vi "AlliGator Send Local Decay Plots.vi"(8 "error in (no error)":errorcluster, 10 "ROI Descriptor":T1 {"Contours"."Type" items=["No Selection", "Point", "Line", "Rectangle", "Oval", "Polygon", "Freehand Region", "Annulus", "Unused2", "Unused3", "Broken Line", "Freehand Line", "Rotated Rectangle"]}, 11 "AlliGator IV DVR in":refnum<data-value>) -> (0 "error out":errorcluster, 3 "AlliGator IV DVR out":refnum<data-value>)   [LabVIEW 2021, in "AlliGator Local Decay Window.lvlib"]
doc: "Gets the data (decay, fit, IRF, residuals and fit parameters) at the selected ROI and sends it to the Local Decay Window for update."
uses:
  AlliGator Local Decay Window.lvlib
  AlliGator Internal Variables v2.ctl
  <vilib>/vision/Image Controls.llb/IMAQ Image.ctl
  AlliGator Gate Image Set.ctl
  AlliGator FLI Dataset Type.ctl
  AlliGator Data Series Type.ctl
  AlliGator Dataset Channel.ctl
  AlliGator Gate Arithmetic.ctl
  AlliGator Displayed Image.ctl
  Image/Named ROI Description.ctl
  AlliGator Decay Metadata v3.ctl
  AlliGator Decay Background Subtraction Info.ctl
  AlliGator Baseline Subtraction Method.ctl
  Graphs/XY Graph/XY Graph Plot Shift Parameters.ctl
  Graphs/XY Graph/XY Graph Plot Shift Method.ctl
  AlliGator Decay Extrapolation Parameters.ctl
  Phasor/Calibration Phasor (m, phi).ctl
  Phasor/Phasor Reference Series.ctl
  Phasor/Phasor Calibration Map v2.ctl
  Phasor/Phasor (g, s).ctl
  AlliGator Raw Phasor Plot Data v4.ctl
  Phasor/Phasor Standard Deviation Options.ctl
  AlliGator Phasor Multi-Harmonic Data.ctl
  Phasor/Phasor Harmonic Data.ctl
  AlliGator Decay Fit Options & Parameters v2.ctl
  Fits/IRF(X)PSED/Decay Fit Options v2.ctl
  Fits/Decay Convolution/Decay Model.ctl
  Fits/Residual Type.ctl
  Fits/IRF(X)PSED/Fit Weights Type.ctl
  Fits/Non-linear Fitting Method v2.ctl
  Fits/Fit Calculation Method.ctl
  Fits/Non-linear Fitting Algorithm.ctl
  AlliGator Decay Fit Parameter Constraints 2.ctl
  Fits/IRF(X)PSED/Decay Fit Parameters In List.ctl
  Fits/IRF(X)PSED/MLE Baseline Offset Type.ctl
  AlliGator Decay Preprocessing Parameters.ctl
  Fits/IRF(X)PSED/Decay Fit Parameters & Derived Quantities List.ctl
  AlliGator Variables List.ctl
  AlliGator Local Decay Graph Window Event Refnum.ctl
  AlliGator Local Decay Fit Results.ctl
  AlliGator Image Profile Plot Data.ctl
  Graphs/XY Graph/XY Plot Data.ctl
  Utilities/Read-Write.ctl
  Variant/Variant to Data/Variant to U16.vi
  Variant/Variant to Data/Variant to Boolean.vi
  AlliGator Globals, Variables & Constants.lvlib
  Graphs/XY Graph/XY Graph Add-Ons.lvlib
  AlliGator Image Profile Window.lvlib
  AlliGator Decay Processing.lvlib
  Time/Time.lvlib
  AlliGator Decay Fit Parameter Map.lvlib
  AlliGator Decay Preprocessing.lvlib
  AlliGator GUI.lvlib
  Utilities/Utilities.lvlib
  Variant/Variant to Data/Variant to Data.lvlib
  Image/Image.lvlib
  Phasor/Phasor.lvlib
  AlliGator Internal Variables.lvlib
  AlliGator Files.lvlib
  AlliGator Phasor Graph.lvlib
  AlliGator Phasor Plot.lvlib
  AlliGator Source Image.lvlib
  Fits/Fits.lvlib
  AlliGator Decay Fit.lvlib
  AlliGator Settings.lvlib
  AlliGator Dual-Channel Datasets.lvlib
panel:
  out "CPU (s)":dbl
  # "see the AlliGator License on the block diagram (Ctrl+E or Window:Show Block Diagram)"
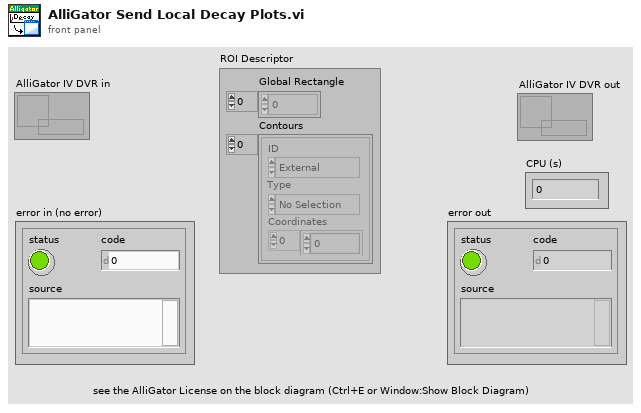
[diagram p1: front panel]
types:
  T1 = typedef "ROI Descriptor" = cluster{"Global Rectangle":i32[], "Contours":cluster{"ID":enum32{"External", "Internal"}, "Type":u32, "Coordinates":i32[]}[]}
  T2 = typedef "AlliGator Local Decay Window.lvlib/AlliGator Local Decay Graph Window Event Refnum.ctl" = refnum<user-event>
  T3 = typedef "AlliGator Globals, Variables & Constants.lvlib/AlliGator Variables List.ctl" = enum16{"---- GUI ----", "Initialization Status", "State Indicators Refnum", "Original AlliGator Menu Items", "Current Action Loop State", "Script in progress", "Playback", "Loop Playback", "Search ROI Used", "Search ROI", "Decay Graph Max Legend Size", "Intensity Graph Max Legend Size", "Decay Statistics Graph Max Legend Size", "Phasor Graph Max Legend Size", "Phasor Ratio Graph Max Legend Size", "Lifetime Graph Max Legend Size", "---- Files ----", "Export Dataset Frames as Individual Files", "Show Batch Export Help Balloons", "Frames in Dataset", "ptu File Frame Start Indices", "Current Frame in Dataset", "Current Frame Timestamp", "------ Python Plugins ------", "Python Plugins Information", "Python Session", "Valid Python Session?", "---- Source Image ----", "Dataset Loaded", "Dataset Metadata", "Dataset Channel", "Dataset Data Description", "Background Dataset Metadata", "Background Dataset Channel", "Background Dataset Data Description", "Background File Subtraction", "Background File Path", "Background File Pile-up Correction", "Background File Pixel Well Capacity", "Background File Scaling Factor", "Source Image ROIs", "Current Source Image ROI", "Source Image ROI Event Refnum", "X_Source Image Display Range", "X_Source Image Palette Information", "Source Image Palette List", "Source Image Scale", "Current Dataset Load Settings", "Source Image:ROI Overlay Color", "---- Image Profile Window ----", "Image Profile:Overlay ROI in Source Image", "Image Profile Window Event Refnum", "Image Profile:IntensityType", "Image Profile:Intensity Average Type", "Image Profile:Intensity-weighted SDV", "Image Profile:Box Profile Type", "Image Profile Window Open", "Image Profile:Plotted Fit Parameter", "X_Type of Displayed Image", "X_Time Gate Slider", "Dataset Path", "Source Image Overlay to Erase", "Is Displayed Image Accumulated", "White Light Image Modified", "Mask Image Modified", "Macrotime Gate Separation", "------ Phasor Graph -------", "Phasor Graph:Show Line", "---- Phasor Plot ---", "Phasor Plot Parameters Changed", "FLI Dataset Modified since last Phasor Plot Calculation", "Phasor Harmonics Data", "Selected Phasor Harmonics", "Phasor Harmonic Manager Event Refnum", "Phasor Plot ROIs", "Current Phasor Plot ROI", "Phasor Plot ROI Event Refnum", "Phasor Plot Image Reference Points", "Phasor Plot Computed", "Phasor Plot Palette Information", "Phasor Plot Palette List", "Phasor Ratio Palette Information", "Phasor Ratio Palette List", "Phasor Image Scale", "Phasor Plot Image Overlay to Erase", "Phasor Plot Image Elements to Update", "Current Phasor Plot Calculation Parameters", "Current Phasor Calibration Options", "Reset Cumulated Phasor Plot", "Phasor Ratio Reference 1", "Phasor Ratio Lifetime Reference 1", "Phasor Ratio Reference 1 Frequency", "Phasor Ratio Reference 2", "Phasor Ratio Lifetime Reference 2", "Phasor Ratio Reference 2 Frequency", "---- Decay Analysis ----", "Number of Selected Decays to Fit", "LS Fit Results", "LAR Fit Results", "BS Fit Results", "Last Decay Max - Min", "Best Fit Parameters", "Best Fit Parameter Names", "Actual Size X", "Actual Size Y", "Binning X", "Binning Y", "Actual # Gates", "Dataset Number", "Gates to...", "Gates Skipped", "Gates to keep", "Gate Step", "Gate Separation", "Reversed Gates", "Pile-up Correction", "Pixel Well Capacity", "Background Subtracted", "Background Subtraction Method", "Background Definition Range", "Background File (deprecated)", "Number of Dataset Accumulated", "Array of Accumulated Dataset Paths", "Do Averaged Datasets", "Destination File Path", "Process Plot Target", "Use 1/D as Phasor Frequency", "---- Decay Fit Parameter Map -----", "Decay Fit Parameter Map Palette Information", "Decay Fit Parameter Map Palette List", "Local Decay Graph Window Event Refnum", "------- Local Decay Window ---------", "Use normalized IRF for convolution", "----- Miscellaneous ----", "Skippable Dialog Windows Status"}
  T4 = typedef "IMAQ Image.ctl" = refnum<image>
  T5 = typedef "Utilities.lvlib/Read-Write.ctl" = enum16{"Read", "Write"}
  T6 = typedef "AlliGator Image Profile Window.lvlib/AlliGator Image Profile Plot Data.ctl" = cluster{"Plot Name":string, "Plot":T7}
  T7 = typedef "XY Graph Add-Ons.lvlib/XY Plot Data.ctl" = cluster{"X Array":dbl[], "Y Array":dbl[]}
  T8 = typedef "AlliGator Internal Variables.lvlib/AlliGator Internal Variables v2.ctl" = cluster{"Displayed Image":T4, "White Light Image":T4, "Mask Image":T4, "ROI Mask Image":T4, "Current Dataset Images 1":T9, "Background Dataset Images 1":T9, "Current Dataset Images 2":T9, "Background Dataset Images 2":T9, "Current Dataset Arithmetic Images":T9, "Accumulated Dataset Images 1":T9, "Accumulated Dataset Images 2":T9, "Accumulated Dataset Arithmetic Images":T9, "Phasor Plot Image":T4, "Decay Fit Parameter Map Image":T4, "Single Data Point Path":path, "White Light Image Path":path, "Mask Image Path":path, "Time-Series Folder":path, "[Time-Series Paths]":path[], "Current Dataset":i32, "Single Dataset Type":T10, "Current Folder":string, "AlliGator Data Series Type":T11, "# Datasets":i32, "Dual-Channel Dataset":bool, "Selected Channel Name":string, "Dataset Channel":T12, "Channel Arithmetic":T13, "Dual-Channel Background Dataset":bool, "Background Channel":T12, "Dual-Channel Accumulated Dataset":bool, "Start Time":dbl, "[Time-Series Timestamps]":dbl[], "[Intensity Corrections]":dbl[], "Time Series Script":bool, "Type of Displayed Image":T14, "Gate Image Slide":u16, "# Gates":i32, "ROIs":T15[], "ROI Decay":cluster{"t Array":dbl[], "I Array":dbl[]}, "Valid Decay":bool, "Decay  Metadata":T16, "Reference Decay Plot Name":string, "Reference Decay":cluster{"t Array":dbl[], "I Array":dbl[]}, "Decay Shift Plot":cluster{"Time Stamps":dbl[], "Decay Shifts":dbl[]}, "[Decays Max Values]":sgl[], "[Decays Min Values]":sgl[], "Calibration Phasor":T22, "Calibration Phasor Series":T23, "Phasor Calibration Map":T24, "Calibration Map MD5 Digest":string, "Last Raw Phasor":T25, "Last Calibrated Phasor":T25, "Last Calibrated Phasor SDV":T25, "Phasor Graph:Phasor Plot":cluster{"g Array":dbl[], "s Array":dbl[]}, "Phasor Graph:Phasor SDV Plot":cluster{"g Array":dbl[], "s Array":dbl[]}, "[Phasor Graph:Raw Phasor Plots]":T26[], "Phasor Plot locked to Ref 1":i32, "[Phasor Plot(s) locked to Ref 1]":i32[], "[Phasor Plot(s) locked to Ref 2]":i32[], "[Pixel Phasors]":T25[], "[[Sum Image]]":dbl[][], "[[CSG Phasors]]":csg[][], "[[Valid Pixel?]]":bool[][], "I/m/phi Dataset":cluster{"I/m/phi Dataset?":bool, "Base Frequency":dbl[unit], "Harmonic Orders":u8[]}, "Multi Phasor Plot Data":T28, "Decay Fit Options & Parameters":T30, "Fit Options: Decay Preprocessing Parameters":T41, "Fit Options: Reference Decay":cluster{"t Array":dbl[], "I Array":dbl[]}, "Is Full Image Parameters Map":bool, "Is Single-Pixels Parameters Map":bool, "NLSF Parameters Map X Resolution":i32, "NLSF Parameters Map Y Resolution":i32, "[Single Decay Fit Parameters]":dbl[], "Fit Model":T32, "[[Multiple Decays Fit Parameters]]":dbl[][], "[[Multiple Decays Fit Parameter SDVs]]":dbl[][], "[[IRFs]]":dbl[][], "IRF Array Time Axis":dbl[], "Decay Array Time Axis":dbl[], "[Decay Fit Parameter Names]":T42[], "[[Phasor Ratios]]":dbl[][], "[[Average Lifetimes]]":dbl[][], "Amplitude Weighted Average Lifetime":bool, "[Decay Sum]":dbl[], "[[User-defined Quantities]]":dbl[][], "User-defined Quantity":string}
  T9 = typedef "AlliGator Internal Variables.lvlib/AlliGator Gate Image Set.ctl" = cluster{"SGL Image Max":T4, "SGL Image Sum":T4, "SGL Gate Images":T4[], "SGL Image Min":T4}
  T10 = typedef "AlliGator Files.lvlib/AlliGator FLI Dataset Type.ctl" = enum16{"HDF5 FLI Dataset", "Gate Image Folder", ".sdt FLI Dataset (Becker & Hickl)", ".ptu FLI Dataset (PicoQuant)", "SS1 FLI Dataset", "SS2 FLI Dataset", "I/m/phi Dataset", ".bin FLI Dataset (PicoQuant Binned)", ".bin FLI Dataset (Piccolo Binned)"}
  T11 = typedef "AlliGator Files.lvlib/AlliGator Data Series Type.ctl" = enum16{"Not a Supported Series", "Gate Images Folder Series", "SwissSPAD 2 Dataset Series", "B&H FLI Dataset Series", "PicoQuant PTU FLI Dataset Series", "PicoQuant BIN FLI Dataset Series", "Piccolo hist BIN FLI Dataset Series", "HDF5 FLI Dataset Series"}
  T12 = typedef "AlliGator Dual-Channel Datasets.lvlib/AlliGator Dataset Channel.ctl" = enum16{"G2", "INT"}
  T13 = typedef "AlliGator Settings.lvlib/AlliGator Gate Arithmetic.ctl" = enum16{"None", "INT-G2", "G2/INT*<INT>", "(1 - G2/INT)*<INT>"}
  T14 = typedef "AlliGator Source Image.lvlib/AlliGator Displayed Image.ctl" = enum16{"Single Gate", "Sum of All Gates", "Max of All Gates", "Min of All Gates", "-", "White Ligth Image", "Mask Image"}
  T15 = typedef "Image.lvlib/Named ROI Description.ctl" = cluster{"ROI Descriptor":T1, "ROI Name":string, "Overlay Color":u32}
  T16 = typedef "AlliGator Phasor Graph.lvlib/AlliGator Decay Metadata v3.ctl" = cluster{"ROI Descriptor":T1, "ROI Center":cluster{"X":i32, "Y":i32}, "Decay Background Subtraction Info":T17, "Decay Reverted":bool, "Decay Smoothened":bool, "Decay Straightened":bool, "Fitted Tau (Decay Straightening)":dbl, "Decay Shift Parameters":T19, "Decay Shifted":bool, "Decay Extrapolated":bool, "Decay Extrapolation Parameters":T21, "Decay Normalized":bool, "Fold Decay":bool, "# Folds":u32}
  T17 = typedef "AlliGator Decay Analysis.lvlib/AlliGator Decay Preprocessing.lvlib/AlliGator Decay Background Subtraction Info.ctl" = cluster{"Laser Period":dbl[unit], "Gate Duration":dbl[unit], "Baseline Subtraction Method":T18, "Background Definition Range":cluster{"Min Gate":dbl[unit], "Max Gate":dbl[unit]}, "Total Intensity w/o Bkgd Subtraction":dbl, "Bkgd-subtracted Intensity (exp)":dbl, "# Data Points":i32, "Background/Gate":dbl, "Fitted Lifetime":dbl[unit], "Bkgd-subtracted Intensity (theo)":dbl}
  T18 = typedef "AlliGator Decay Analysis.lvlib/AlliGator Decay Preprocessing.lvlib/AlliGator Baseline Subtraction Method.ctl" = enum16{"Mean", "Min", "Square Gated Single-Exponential", "File", "Constant"}
  T19 = typedef "XY Graph Add-Ons.lvlib/XY Graph Plot Shift Parameters.ctl" = cluster{"Type":T20, "Shift":dbl[unit], "Threshold":dbl, "Rotate":bool}
  T20 = typedef "XY Graph Add-Ons.lvlib/XY Graph Plot Shift Method.ctl" = enum16{"Default", "CFD", "Threshold", "Cross-Correlation"}
  T21 = typedef "AlliGator Decay Analysis.lvlib/AlliGator Decay Preprocessing.lvlib/AlliGator Decay Extrapolation Parameters.ctl" = cluster{"Additional Points":u32, "Head Fraction":dbl, "Fitted Tau":dbl, "Use Periodicity":bool, "Use Cursors":bool, "Tail Fraction":dbl}
  T22 = typedef "Phasor.lvlib/Calibration Phasor (m, phi).ctl" = cluster{"m":dbl, "phi":dbl, "Phasor Frequency":dbl[unit], "Reference Lifetime":dbl[unit]}
  T23 = typedef "Phasor.lvlib/Phasor Reference Series.ctl" = cluster{"m Array":dbl[], "phi Array":dbl[], "Phasor Frequency":dbl[unit], "Calibration Lifetime":dbl[unit]}
  T24 = typedef "Phasor.lvlib/Phasor Calibration Map v2.ctl" = cluster{"Phasor Frequency":dbl[unit], "Calibration Lifetime":dbl[unit], "ROI Centers":cluster{"X":i32, "Y":i32}[], "ROI Descriptors":T1[], "Map Resolution X":i32, "Map Resolution Y":i32, "z Array":cdb[]}
  T25 = typedef "Phasor.lvlib/Phasor (g, s).ctl" = cluster{"g":dbl, "s":dbl}
  T26 = typedef "AlliGator Phasor Graph.lvlib/AlliGator Raw Phasor Plot Data v4.ctl" = cluster{"Phasor Plot Name":string, "Raw Phasor Plot":T25[], "Phasor Frequency":dbl[unit], "[Decay Metadata]":T16[], "Raw Phasor Plot SDV":T25[], "Phasor SDV Options":T27, "[Calibration Phasor]":T22[]}
  T27 = typedef "Phasor.lvlib/Phasor Standard Deviation Options.ctl" = cluster{"Compute Estimated SDV":bool, "# Replicas":u32, "Use Estimated Average Phasor":bool}
  T28 = typedef "AlliGator Phasor Plot.lvlib/AlliGator Phasor Multi-Harmonic Data.ctl" = cluster{"Base Frequency":dbl[unit], "# Harmonics":u8, "Harmonic Orders":u8[], "Phasor Plot Settings Checksum":u64, "Phasor Harmonic Data Array":T29[]}
  T29 = typedef "Phasor.lvlib/Phasor Harmonic Data.ctl" = cluster{"Phasor Harmonic Name":string, "Phasor Plot Settings Checksum":u64, "Phasor Frequency":dbl[unit], "Base Frequency":dbl[unit], "Harmonic Order":u8, "Phasor Plot Parameters":string, "Phasor Array [[CSG]]":csg[][], "Dataset File Path":path}
  T30 = typedef "AlliGator Decay Fit Parameter Map.lvlib/AlliGator Decay Fit Options & Parameters v2.ctl" = cluster{"SYNC Period":dbl[unit], "Fit Options":T31, "Fit Parameter Constraints":T38[], "MLE Baseline Offset":dbl, "MLE Baseline Offset Type":T40}
  T31 = typedef "Fits.lvlib/Decay Fit Options v2.ctl" = cluster{"Show Fit Residuals":bool, "Fit Model":T32, "Residual Type":T33, "Max Decay Percentile":dbl, "Min Decay Percentile":dbl, "Show Full Decay":bool, "Weights":T34, "Fitting Method":T35, "Compute Parameter Uncertainties":bool, "Periodic Boundaries":bool, "Model Calculation":T36, "Period":dbl[unit], "Termination Criteria":cluster{"Max Iterations":i32, "Max Function Calls":i32, "Max Time":dbl[unit], "Function Tolerance":dbl, "Parameter Tolerance":dbl, "Gradient Tolerance":dbl, "Min Lambda":dbl, "Max Lambda":dbl, "Initial Tick Count":u32}, "Offset Resolution":dbl[unit], "Use Local IRF":bool, "Fitting Algorithm":T37}
  T32 = typedef "Fits.lvlib/Decay Model.ctl" = enum16{"1-Exponential", "2-Exponentials"}
  T33 = typedef "Fits.lvlib/Residual Type.ctl" = enum16{"Standard", "Normalized", "Reduced"}
  T34 = typedef "Fits.lvlib/Fit Weights Type.ctl" = enum16{"Unweighted", "1/Variance", "Best of All"}
  T35 = typedef "Fits.lvlib/Non-linear Fitting Method v2.ctl" = enum16{"Least Square", "Least Absolute Residual", "Bisquare", "MLE", "-", "Best of All"}
  T36 = typedef "Fits.lvlib/Fit Calculation Method.ctl" = enum16{"Simulation", "Convolution", "Integration"}
  T37 = typedef "Fits.lvlib/Non-linear Fitting Algorithm.ctl" = enum16{"Levenberg-Marquardt", "Trust-Region Dogleg"}
  T38 = typedef "AlliGator Decay Analysis.lvlib/AlliGator Decay Fit.lvlib/AlliGator Decay Fit Parameter Constraints 2.ctl" = cluster{"Fit Parameter":T39, "Min Value":dbl, "Max Value":dbl, "Global":bool, "Used":bool}
  T39 = typedef "Fits.lvlib/Decay Fit Parameters In List.ctl" = enum16{"Offset", "Baseline", "A_1", "tau_1", "A_2", "tau_2"}
  T40 = typedef "Fits.lvlib/MLE Baseline Offset Type.ctl" = enum32{"Absolute", "Percentage"}
  T41 = typedef "AlliGator Decay Analysis.lvlib/AlliGator Decay Preprocessing.lvlib/AlliGator Decay Preprocessing Parameters.ctl" = cluster{"Background Subtraction":bool, "Straighten Decay":bool, "Reverse Gates":bool, "1-Normalized Decay":bool, "Smoothen Decay":bool, "Smoothing Parameter":dbl, "Shift Decay":bool, "Decay Shift Parameters":T19, "Extrapolate Decay":bool, "Additional Points":u32, "Head Fraction":dbl, "Pixel-Normalize Decay":bool, "Use Periodicity":bool, "Use Cursors":bool, "Tail Fraction":dbl, "Use Decay Pre-Processing":bool, "Fold Decay":bool, "# Folds":u32, "[0-1]-Normalized Decay":bool}
  T42 = typedef "Fits.lvlib/Decay Fit Parameters & Derived Quantities List.ctl" = enum16{"Offset", "Baseline", "A_1", "tau_1", "A_2", "tau_2", "<tau>_a", "f1_a", "f2_a", "<tau>_i", "f1_i", "f2_i", "-", "R^2", "Chi^2"}
  T43 = cluster{"IRF Array Time Axis":dbl[], "[[IRFs]]":dbl[]}
  T44 = cluster{"t Axis":dbl[], "ROI Intensity Array":dbl[]}
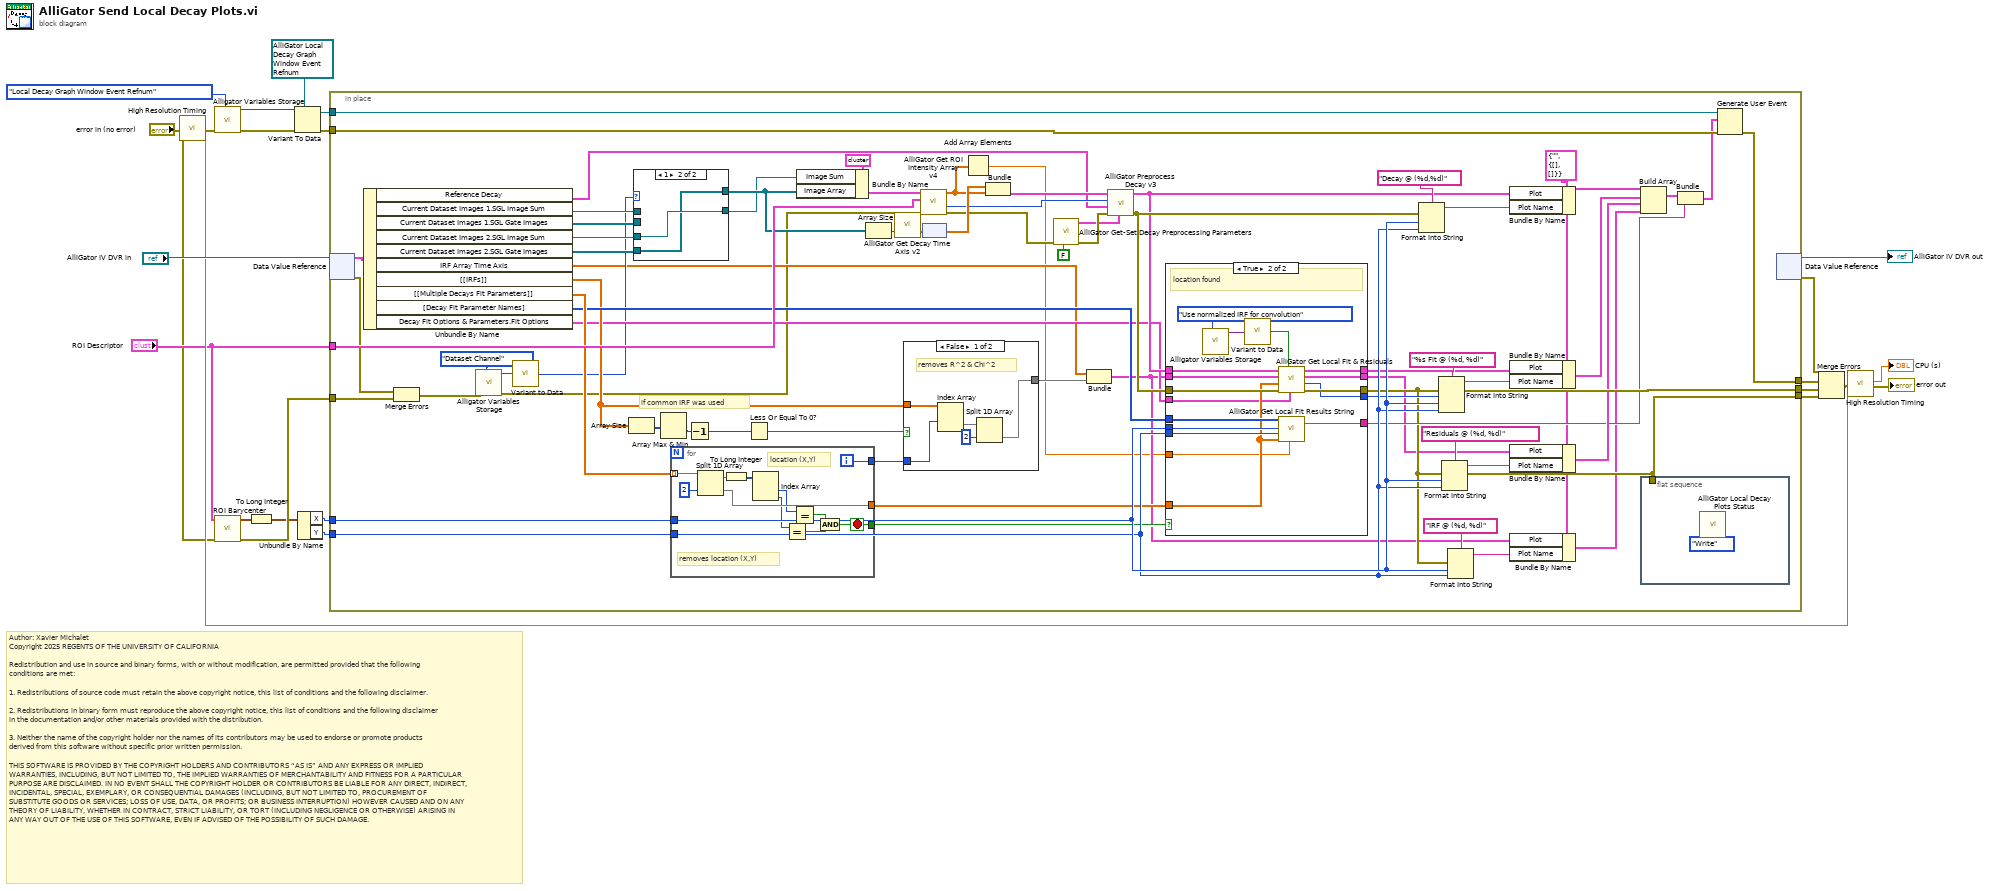
[diagram p0: block diagram]
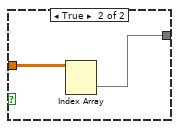
[diagram p3: hidden frame]
diagram:
  # "Author: Xavier Michalet\nCopyright 2025 REGENTS OF THE UNIVERSITY OF CALIFORNIA\n\nRedistribution and use in source and binary forms, with or without modification, are permitted provided that the following conditions are met:\n\n1. Redistributions of source code must retain the above copyright notice, this list of conditions and the following disclaimer.\n\n2. Redistributions in binary form must reproduce the above copyright notice, this list of conditions and the following disclaimer in the documentation and/or other materials provided with the distribution.\n\n3. Neither the name of the copyright holder nor the names of its contributors may be used to endorse or promote products derived from this software without specific prior written permission.\n\nTHIS SOFTWARE IS PROVIDED BY THE COPYRIGHT HOLDERS AND CONTRIBUTORS “AS IS” AND ANY EXPRESS OR IMPLIED WARRANTIES, INCLUDING, BUT NOT LIMITED TO, THE IMPLIED WARRANTIES OF MERCHANTABILITY AND FITNESS FOR A PARTICULAR PURPOSE ARE DISCLAIMED. IN NO EVENT SHALL THE COPYRIGHT HOLDER OR CONTRIBUTORS BE LIABLE FOR ANY DIRECT, INDIRECT, INCIDENTAL, SPECIAL, EXEMPLARY, OR CONSEQUENTIAL DAMAGES (INCLUDING, BUT NOT LIMITED TO, PROCUREMENT OF SUBSTITUTE GOODS OR SERVICES; LOSS OF USE, DATA, OR PROFITS; OR BUSINESS INTERRUPTION) HOWEVER CAUSED AND ON ANY THEORY OF LIABILITY, WHETHER IN CONTRACT, STRICT LIABILITY, OR TORT (INCLUDING NEGLIGENCE OR OTHERWISE) ARISING IN ANY WAY OUT OF THE USE OF THIS SOFTWARE, EVEN IF ADVISED OF THE POSSIBILITY OF SUCH DAMAGE."
  n1 = call "High Resolution Timing.vi"("Error In"="error in (no error)") -> ("elapsed (relative) seconds"=w10:dbl, "Error Out"=w13:errorcluster)  [unwired: 16 in, 1 out]
  n2 = call "Alligator Variables Storage.vi"("AlliGator Variable"=AlliGator_Variables_List."Local Decay Graph Window Event Refnum" ("Alligator Variable"), "Error In"=w13) -> ("Error Out"=w21:errorcluster, "Data out"=w19:variant)  [unwired: 7 in, 1 out]
  n3 = call "ROI Barycenter.vi"("Error In"="error in (no error)", "ROI Descriptor in"="ROI Descriptor") -> ("Error Out"=w2:errorcluster, "ROI Center"=w5:cluster{"X":dbl, "Y":dbl})  [unwired: 8 in]
  n4 = To Long Integer(number=w5) -> (32bit integer=w1:cluster{"X":i32, "Y":i32})
  n5 = Variant To Data(error in=w21, type=T2 refnum ("Local Decay Graph Window Event Refnum"), Variant=w19) -> (data=w17:T2, error out=w20:errorcluster)
  n6 = Unbundle By Name(w1) -> ("X"=w15:i32, "Y"=w14:i32)
  n7 = in-place {
    in-place-border: w20 -> [w89]
    in-place-border: w17 -> [w95]
    in-place-border: [w94] -> w16
    in-place-border: w15 -> [w93]
    in-place-border: w14 -> [w92]
    in-place-border: "ROI Descriptor" -> [w91]
    in-place-border: [w88] -> w8
    in-place-border: [w87] -> w7
    in-place-border: w2 -> [w86]
    w33 = T6 {"Plot Name"="", "Plot"={"X Array"=[], "Y Array"=[]}} ("Plot Data")
    # "if common IRF was used"
    n8 = in-place-dvr #1("AlliGator IV DVR in") -> (w96:T8, w90:errorcluster)
    n9 = Unbundle By Name(w96) -> ("Reference Decay"=w27:cluster{"t Array":dbl[], "I Array":dbl[]}, "Current Dataset Images 1.SGL Image Sum"=w49:T4, "Current Dataset Images 1.SGL Gate Images"=w52:T4[], "Current Dataset Images 2.SGL Image Sum"=w48:T4, "Current Dataset Images 2.SGL Gate Images"=w51:T4[], "IRF Array Time Axis"=w35:dbl[], "[[IRFs]]"=w42:dbl[][], "[[Multiple Decays Fit Parameters]]"=w70:dbl[][], "[Decay Fit Parameter Names]"=w67:T42[], "Decay Fit Options & Parameters.Fit Options"=w39:T31)
    n10 = Merge Errors(w90, w86) -> (w28:errorcluster)
    n11 = call "Alligator Variables Storage.vi"("AlliGator Variable"=AlliGator_Variables_List."Dataset Channel" ("Alligator Variable"), "Error In"=w28) -> ("Error Out"=w29:errorcluster, "Data out"=w37:variant)  [unwired: 7 in, 1 out]
    n12 = call-poly "Variant to Data.vi"("Variant"=w37) -> ("U16 Value"=w36:u16)  [unwired: 8 in]
    n13 = Array Size(array=w42) -> (size(s)=w46:i32[])
    n14 = case shown="1" w36 {
      tunnel: [w99 w101] -> w47
      tunnel: w48 -> [_ w101]
      tunnel: w51 -> [_ w100]
      tunnel: [w98 w100] -> w50
      tunnel: w49 -> [w99 _]
      tunnel: w52 -> [w98 _]
      frame 0, Default {
      }
      frame 1 {
      }
    }
    n15 = Array Max & Min(array=w46) -> (min value=w45:i32)  [unwired: 3 out]
    n16 = for {
      tunnel: w70 -> [w139] mode=indexing
      tunnel: w93 -> [w138]
      tunnel: w92 -> [w137]
      tunnel: [w136] -> w76
      tunnel: [w135] -> w71
      tunnel: [w129] -> w41
      i -> [w129]
      stop <- w136 stop-if-true
      # "location (X,Y)"
      # "removes location (X,Y)"
      n17 = Split 1D Array(array=w139, index=2) -> (first subarray=w128:dbl[], second subarray=w135:dbl[])
      n18 = To Long Integer(number=w128) -> (32bit integer=w127:i32[])
      n19 = Index Array(array=w127) -> (element #1=w133:i32, element #2=w132:i32)  [unwired: 2 in]
      n20 = Equal?(x=w132, y=w137) -> (x = y?=w130:bool)
      n21 = Equal?(x=w133, y=w138) -> (x = y?=w131:bool)
      n22 = And(x=w131, y=w130) -> (x .and. y?=w136:bool)
    }
    n23 = Decrement(x=w45) -> (x-1=w44:i32)
    n24 = Less Or Equal To 0?(x=w44) -> (x <= 0?=w43:bool)
    n25 = Bundle By Name(cluster=cluster{"Image Sum":T4, "Image Array":T4[]} {"Image Sum"=refnum, "Image Array"=[]} ("Images"), "Image Sum"=w47, "Image Array"=w50) -> (w74:cluster{"Image Sum":T4, "Image Array":T4[]})
    n26 = Array Size(array=w50) -> (size(s)=w73:i32)
    n27 = call "AlliGator Get Decay Time Axis v2.vi"("Number of Gates"=w73) -> ("t Array"=w72:dbl[unit][])  [unwired: 14 in]
    n28 = case shown="False" w43 {
      tunnel: w42 -> [w106 w108]
      tunnel: [w102 w107] -> w34
      tunnel: w41 -> [w105 _]
      frame False {
        # "removes R^2 & Chi^2"
        n29 = Index Array(array=w106, index (row)=w105) -> (element=w104:dbl[])  [unwired: 1 in]
        n30 = Split 1D Array(array=w104, index=2) -> (second subarray=w102:dbl[])  [unwired: 1 out]
      }
      frame True {
        n31 = Index Array(array=w108) -> (element=w107:dbl[])  [unwired: 2 in]
      }
    }
    n32 = call "AlliGator Get ROI Intensity Array v4.vi"("error in (no error)"=w29, "ROI Descriptor"=w91, "Images"=w74) -> ("Error Out"=w60:errorcluster, "# Valid Pixels"=w58:i32, "ROI Intensity Array"=w26:dbl[])  [unwired: 3 in, 3 out]
    n33 = node(w72) -> (w69:dbl[])
    n34 = Add Array Elements(numeric array=w26) -> (sum=w25:dbl)
    n35 = Bundle(w69, "ROI Intensity Array"=w26) -> (w57:cluster{dbl[], "ROI Intensity Array":dbl[]})  [unwired: 1 in]
    n36 = call "AlliGator Get-Set Decay Preprocessing Parameters.vi"("Get (F)/Set"=FALSE, "Error In"=w60) -> ("Error Out"=w59:errorcluster, "Decay Preprocessing Parameters out"=w55:T41)  [unwired: 8 in]
    n37 = Bundle("IRF Array Time Axis"=w35, "[[IRFs]]"=w34) -> (w30:T43)  [unwired: 1 in]
    n38 = call "AlliGator Preprocess Decay v3.vi"("Decay Preprocessing Parameters"=w55, "Error In"=w59, "Time-Gated Reference Decay"=w27, "# Pixels"=w58, "Decay (in)"=w57) -> ("Error Out"=w56:errorcluster, "Decay (out)"=w53:T44)  [unwired: 3 in, 2 out]
    n39 = case shown="True" w76 {
      tunnel: w71 -> [_ w118]
      tunnel: w56 -> [w109 w126]
      tunnel: [w109 w125] -> w40
      tunnel: w53 -> [_ w124]
      tunnel: [_ w123] -> w68
      tunnel: w67 -> [_ w122]
      tunnel: w93 -> [_ w121]
      tunnel: w92 -> [_ w120]
      tunnel: [_ w119] -> w65
      tunnel: w39 -> [_ w117]
      tunnel: w30 -> [_ w116]
      tunnel: [_ w115] -> w32
      tunnel: [_ w114] -> w31
      tunnel: w25 -> [_ w110]
      frame False {
        # "Not a valid location"
      }
      frame True {
        # "location found"
        n40 = call "Alligator Variables Storage.vi"("AlliGator Variable"=AlliGator_Variables_List."Use normalized IRF for convolution") -> ("Data out"=w113:variant)  [unwired: 8 in, 2 out]
        n41 = call-poly "Variant to Data.vi"("Variant"=w113) -> ("Value"=w111:bool)  [unwired: 8 in]
        n42 = call "AlliGator Get Local Fit & Residuals.vi"("Fit Options"=w117, "Use Normalized IRF (T)"=w111, "Error In"=w126, "All Fit Parameters (w tau)"=w118, "IRF"=w116, "Decay Plot"=w124) -> ("Error Out"=w125:errorcluster, "Fit Model"=w123:T32, "Residual Plot"=w114:cluster{"X Array":dbl[], "Y Array":dbl[]}, "Fit Plot"=w115:cluster{"X Array":dbl[], "Y Array":dbl[]})  [unwired: 2 in]
        n43 = call "AlliGator Get Local Fit Results String.vi"("Decay Sum"=w110, "Parameters"=w118, "Y"=w120, "X"=w121, "[Decay Fit Parameter Name]"=w122) -> ("Fit Results String"=w119:string)  [unwired: 6 in]
      }
    }
    n44 = Format Into String(format string="Decay @ (%d,%d)" ("Plot Name"), error in=w56, w93, w92) -> (resulting string=w82:string)  [unwired: 1 in, 1 out]
    n45 = Format Into String(format string="%s Fit @ (%d, %d)" ("Plot Name"), error in=w40, w68, w93, w92) -> (resulting string=w79:string, error out=w88:errorcluster)  [unwired: 1 in]
    n46 = Format Into String(format string="Residuals @ (%d, %d)" ("Plot Name"), error in=w40, w93, w92) -> (resulting string=w77:string, error out=w87:errorcluster)  [unwired: 1 in]
    n47 = Format Into String(format string="IRF @ (%d, %d)" ("Plot Name"), error in=w40, w93, w92) -> (resulting string=w62:string)  [unwired: 1 in, 1 out]
    n48 = Bundle By Name(cluster=w33, "Plot"=w53, "Plot Name"=w82) -> (w85:T6)
    n49 = Bundle By Name(cluster=w33, "Plot"=w32, "Plot Name"=w79) -> (w84:T6)
    n50 = Bundle By Name(cluster=w33, "Plot"=w31, "Plot Name"=w77) -> (w83:T6)
    n51 = Bundle By Name(cluster=w33, "Plot"=w30, "Plot Name"=w62) -> (w61:T6)
    n52 = Build Array(w85, w84, w83, w61) -> (w66:T6[])
    n53 = flat-sequence {
      tunnel: w87 -> [_]
      frame #0 {
        n54 = call "AlliGator Local Decay Plots Status.vi"("Read/Write"=Read-Write."Write") -> ()  [unwired: 8 in, 1 out]
      }
    }
    n55 = Bundle(w66, "Fit Results String"=w65) -> (w64:cluster{T6[], "Fit Results String":string})  [unwired: 1 in]
    n56 = Generate User Event(user event=w95, event data cluster=w64, error in=w89) -> (error out=w94:errorcluster)  [unwired: 1 in, 1 out]
    n57 = in-place-dvr #1() -> (→"AlliGator IV DVR out":refnum<data-value>, w6:errorcluster)  [unwired: 1 in]
  }
  n58 = Merge Errors(w6, w16, w8, w7) -> (w12:errorcluster)
  n59 = call "High Resolution Timing.vi"("relative seconds (NaN)"=w10, "Error In"=w12) -> ("elapsed (relative) seconds"=→"CPU (s)":dbl, "Error Out"=→"error out":errorcluster)  [unwired: 15 in, 1 out]
